vi "Pre Launch Init.vi"(11 "Shaker Controller in":refnum<class "Shaker Controller.lvclass">) -> (0 "error out":errorcluster, 3 "Shaker Controller out":refnum<class "Shaker Controller.lvclass">)   [LabVIEW 2020, in "Shaker Controller.lvlib" / "Shaker Controller.lvclass"]
doc: "(<B>Filename</B>: Actor Framework.lvlib:Actor.lvclass:Pre Launch Init.vi)\n\nDefines behavior that occurs after the Launch Nested Actor method is invoked but before the actor's Actor Core method begins running.\n\nBy default, this method does nothing. A descendant class may override it to define behavior."
uses:
  Shaker Controller.lvclass
  _Abstract Classes/Abstract Shake Monitor/Abstract Shake Monitor.lvclass
  _Abstract Classes/Abstract Shaker/Abstract Shaker.lvclass
  Shaker Controller.lvclass/Shaker Controller.ctl
  <vilib>/MGI/Monitored Actor/Monitored Actor/Monitored Actor/Monitored Actor.lvclass
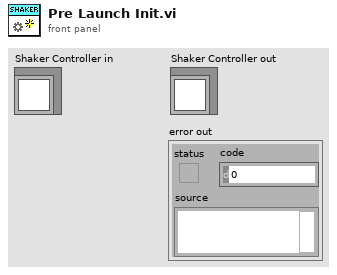
[diagram p1: front panel]
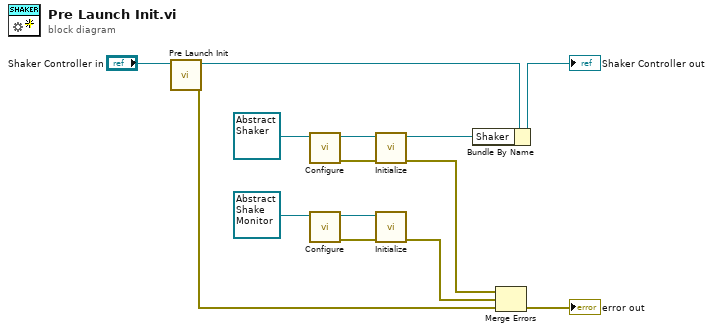
[diagram p0: block diagram]
diagram:
  n1 = call-parent "Pre Launch Init.vi"("Monitored Actor in"="Shaker Controller in") -> ("error out"=w1:errorcluster, "Monitored Actor out"=w13:refnum<class "Shaker Controller.lvclass">)  [unwired: 9 in]
  n2 = call-dynamic "Configure.vi"("Abstract Shaker in"=refnum<class "Abstract Shaker.lvclass"> refnum) -> ("error out"=w8:errorcluster, "Abstract Shaker out"=w11:refnum<class "Abstract Shaker.lvclass">)  [unwired: 9 in]
  n3 = call-dynamic "Configure.vi"("Abstract Shake Monitor in"=refnum<class "Abstract Shake Monitor.lvclass"> refnum ("Shaker Controller.lvlib:Abstract Shake Monitor.lvclass")) -> ("error out"=w6:errorcluster, "Abstract Shake Monitor out"=w7:refnum<class "Abstract Shake Monitor.lvclass">)  [unwired: 9 in]
  n4 = call-dynamic "Initialize.vi"("error in (no error)"=w8, "Abstract Shaker in"=w11) -> ("error out"=w3:errorcluster, "Abstract Shaker out"=w10:refnum<class "Abstract Shaker.lvclass">)  [unwired: 8 in]
  n5 = call-dynamic "Initialize.vi"("error in (no error)"=w6, "Abstract Shake Monitor in"=w7) -> ("error out"=w2:errorcluster)  [unwired: 8 in, 1 out]
  n6 = Bundle By Name(cluster=w13, "Shaker"=w10) -> (→"Shaker Controller out":refnum<class "Shaker Controller.lvclass">)
  n7 = Merge Errors(w3, w2, w1) -> (→"error out":errorcluster)
